vi "acquire multi waves by LAN subvi.vi"(0 "TCP Network Connection in":refnum<k5>, 5 "WFGraph Refnum":refnum<vi>, 7 "data in":string, 9 "data in":string, 11 "error in (no error)":errorcluster) -> (2 "CH1 SCALE":string, 3 "CH1 VOLTS/DIV":string, 4 "CH2 VOLTS/DIV":string, 6 "CH2 SCALE":string, 8 "CH2 PROBE":string, 10 "Waveform Graph":i32[][](graph), 13 "CH1 PROBE":string, 14 "CH2":string)   [LabVIEW 2013]
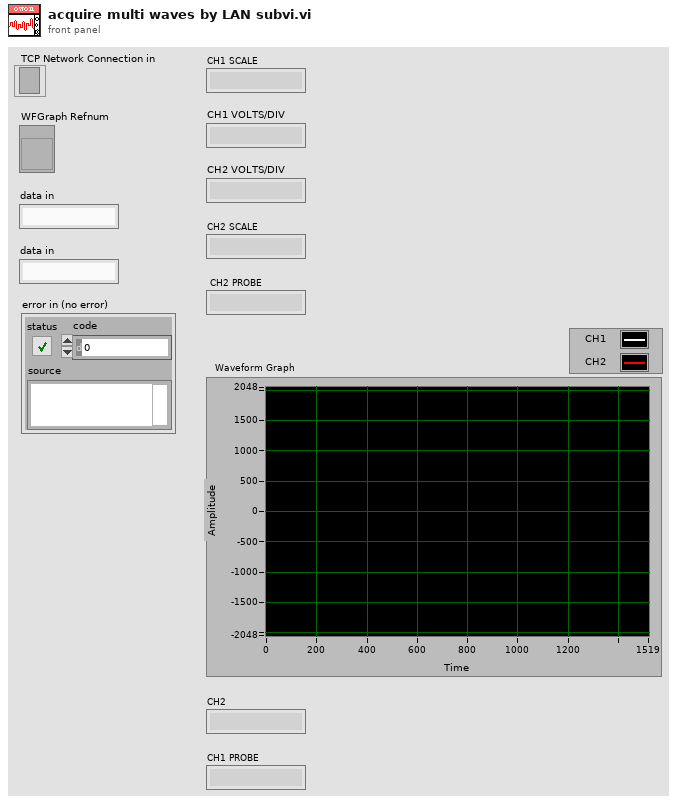
[diagram p1: front panel]
types:
  T1 = enum16{"Standard", "Buffered", "CRLF", "Immediate"}
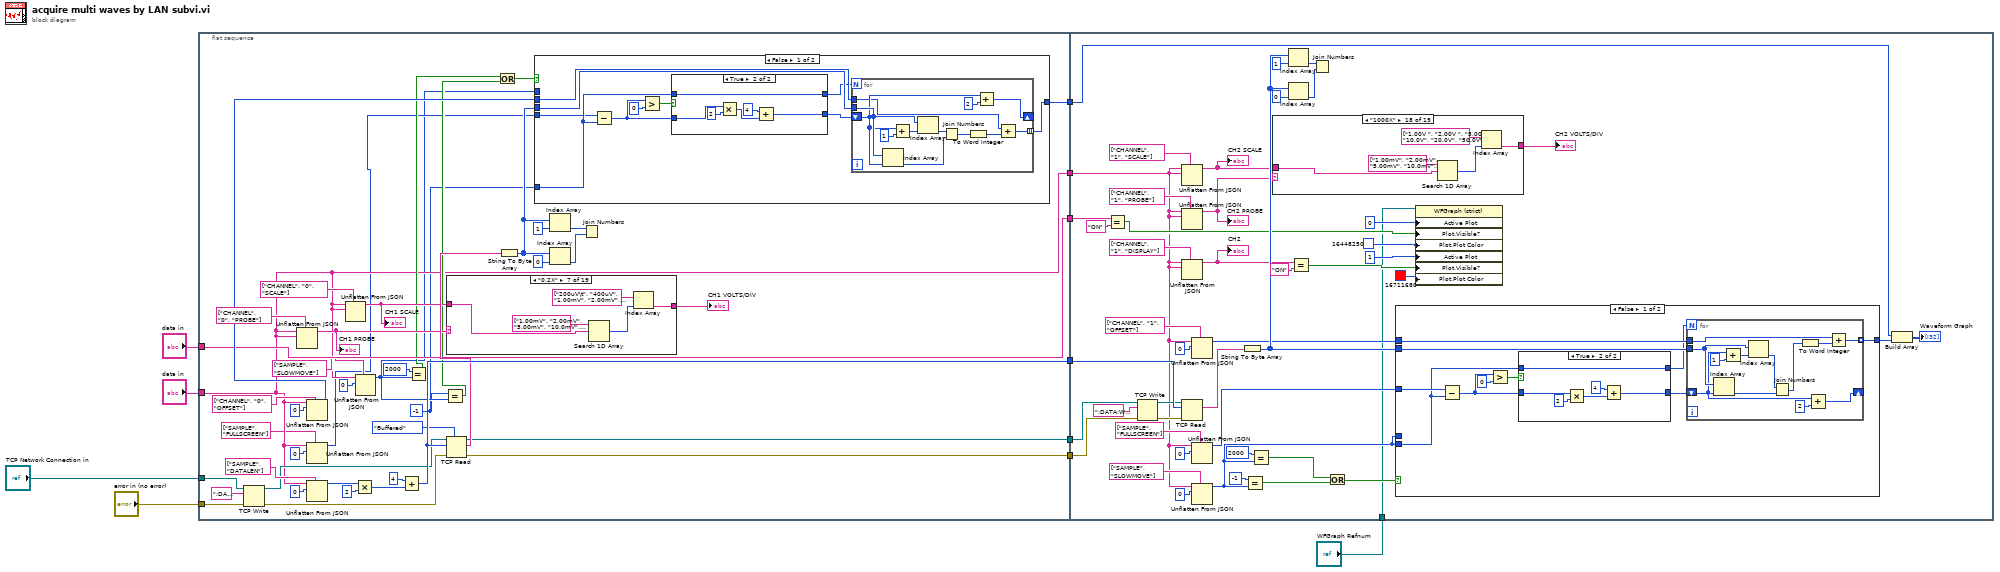
[diagram p0: block diagram]
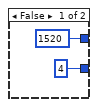
[diagram p2: hidden frame]
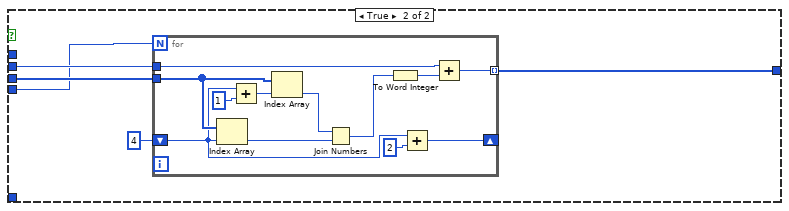
[diagram p3: hidden frame]
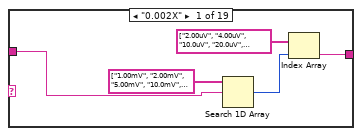
[diagram p4: hidden frame]
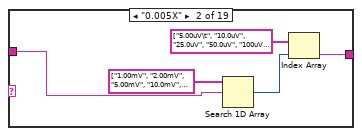
[diagram p5: hidden frame]
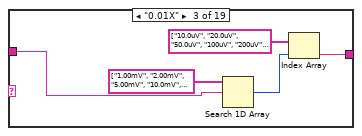
[diagram p6: hidden frame]
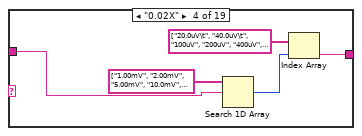
[diagram p7: hidden frame]
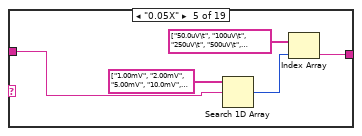
[diagram p8: hidden frame]
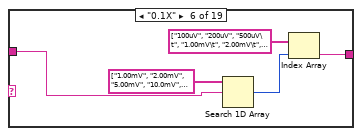
[diagram p9: hidden frame]
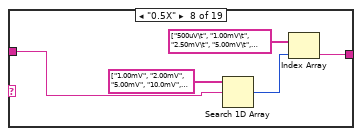
[diagram p10: hidden frame]
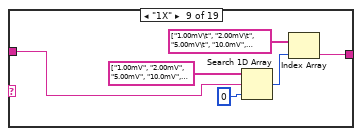
[diagram p11: hidden frame]
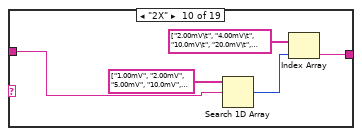
[diagram p12: hidden frame]
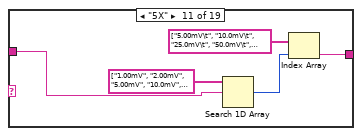
[diagram p13: hidden frame]
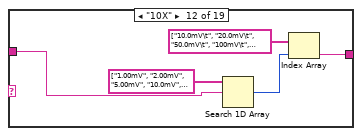
[diagram p14: hidden frame]
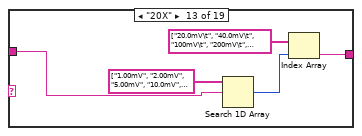
[diagram p15: hidden frame]
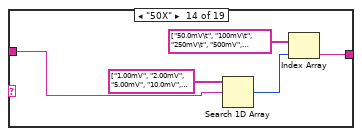
[diagram p16: hidden frame]
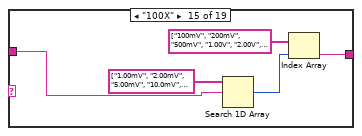
[diagram p17: hidden frame]
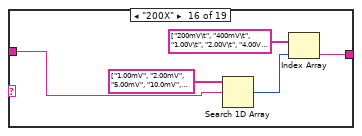
[diagram p18: hidden frame]
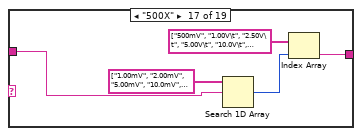
[diagram p19: hidden frame]
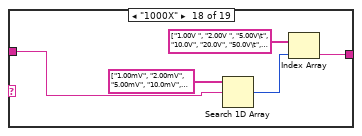
[diagram p20: hidden frame]
diagram:
  n1 = flat-sequence {
    tunnel: [w17] -> w9
    tunnel: [w34] -> w10
    tunnel: [w38] -> w11
    tunnel: "error in (no error)" -> [w36]
    tunnel: "data in" -> [w17]
    tunnel: "TCP Network Connection in" -> [w35]
    tunnel: [w29] -> w8
    tunnel: [w28] -> w7
    tunnel: [w24] -> w6
    tunnel: "data in" -> [w24]
    tunnel: w11 -> [w211]
    tunnel: w10 -> [w230]
    tunnel: w9 -> [w201]
    tunnel: w8 -> [w226]
    tunnel: w7 -> [w225]
    tunnel: w6 -> [w220]
    tunnel: "WFGraph Refnum" -> [w198]
    frame #0 {
      w12 = -1 ("x")
      n2 = TCP Write(connection ID=w35, data in=":DATA:WAVE:SCREEN:CH1?" ("ID Query"), error in (no error)=w36) -> (connection ID out=w33:refnum<k5>, error out=w32:errorcluster)  [unwired: 1 in, 1 out]
      n3 = Unflatten From JSON(path=string[] ["CHANNEL", "0", "PROBE"], JSON string=w17, type and defaults=w17) -> (value=w27:string)  [unwired: 4 in, 1 out]
      "CH1 PROBE" <- w27
      n4 = Unflatten From JSON(path=string[] ["CHANNEL", "0", "OFFSET"], JSON string=w17, type and defaults=0) -> (value=w45:i32)  [unwired: 4 in, 1 out]
      n5 = Unflatten From JSON(path=string[] ["SAMPLE", "FULLSCREEN"], JSON string=w17, type and defaults=0) -> (value=w14:i32)  [unwired: 4 in, 1 out]
      n6 = Unflatten From JSON(path=string[] ["SAMPLE", "DATALEN"], JSON string=w17, type and defaults=0) -> (value=w42:i32)  [unwired: 4 in, 1 out]
      n7 = Unflatten From JSON(path=string[] ["CHANNEL", "0", "SCALE"], JSON string=w17, type and defaults=w17) -> (value=w26:string)  [unwired: 4 in, 1 out]
      "CH1 SCALE" <- w26
      n8 = Multiply(x=w42, y=2) -> (x*y=w40:i32)
      n9 = Unflatten From JSON(path=string[] ["SAMPLE", "SLOWMOVE"], JSON string=w17, type and defaults=0) -> (value=w13:i32)  [unwired: 4 in, 1 out]
      n10 = Add(x=4, y=w40) -> (x+y=w34:i32)
      n11 = Equal?(x=2000, y=w13) -> (x = y?=w19:bool)
      n12 = Equal?(x=w12, y=w13) -> (x = y?=w20:bool)
      n13 = case shown="\"0.2X\"" w27 {
        tunnel: w26 -> [w105 w110 w115 w120 w125 w130 w135 w140 w145 w151 w156 w161 w166 w171 w176 w181 w186 w191 w197]
        tunnel: [w104 w109 w114 w119 w124 w129 w134 w139 w144 w150 w155 w160 w165 w170 w175 w180 w185 w190 w194] -> w25
        frame "0.002X" {
          n14 = Search 1D Array(1D array=string[] ["1.00mV", "2.00mV", "5.00mV", "10.0mV", "20.0mV", "50.0mV", "100mV", "200mV", "500mV", "1.00V", "2.00V", "5.00V", "10.0V", "20.0V"], element=w105) -> (index of element=w106:i32)  [unwired: 1 in]
          n15 = Index Array(array=string[] ["2.00uV", "4.00uV", "10.0uV", "20.0uV", "50.0uV", "100uV", "200uV", "400uV", "1.00mV", "2.00mV\t", "4.00mV", "10.0mV", "20.0mV", "40.0mV"], index=w106) -> (element=w104:string)
        }
        frame "0.005X" {
          n16 = Search 1D Array(1D array=string[] ["1.00mV", "2.00mV", "5.00mV", "10.0mV", "20.0mV", "50.0mV", "100mV", "200mV", "500mV", "1.00V", "2.00V", "5.00V", "10.0V", "20.0V"], element=w110) -> (index of element=w111:i32)  [unwired: 1 in]
          n17 = Index Array(array=string[] ["5.00uV\t", "10.0uV", "25.0uV", "50.0uV", "100uV", "250uV", "500uV", "1.00mV\t", "2.50mV", "5.00mV", "10.0mV", "25.0mV", "50.0mV", "100mV"], index=w111) -> (element=w109:string)
        }
        frame "0.01X" {
          n18 = Search 1D Array(1D array=string[] ["1.00mV", "2.00mV", "5.00mV", "10.0mV", "20.0mV", "50.0mV", "100mV", "200mV", "500mV", "1.00V", "2.00V", "5.00V", "10.0V", "20.0V"], element=w115) -> (index of element=w116:i32)  [unwired: 1 in]
          n19 = Index Array(array=string[] ["10.0uV", "20.0uV", "50.0uV", "100uV", "200uV", "500uV", "1.00mV\t", "2.00mV\t", "5.00mV", "10.0mV\t", "20.0mV\t", "50.0mV", "100mV", "200mV"], index=w116) -> (element=w114:string)
        }
        frame "0.02X" {
          n20 = Search 1D Array(1D array=string[] ["1.00mV", "2.00mV", "5.00mV", "10.0mV", "20.0mV", "50.0mV", "100mV", "200mV", "500mV", "1.00V", "2.00V", "5.00V", "10.0V", "20.0V"], element=w120) -> (index of element=w121:i32)  [unwired: 1 in]
          n21 = Index Array(array=string[] ["20.0uV\t", "40.0uV\t", "100uV", "200uV", "400uV", "1.00mV", "2.00mV", "4.00mV", "10.0mV", "20.0mV", "40.0mV", "100mV", "200mV", "400mV"], index=w121) -> (element=w119:string)
        }
        frame "0.05X" {
          n22 = Search 1D Array(1D array=string[] ["1.00mV", "2.00mV", "5.00mV", "10.0mV", "20.0mV", "50.0mV", "100mV", "200mV", "500mV", "1.00V", "2.00V", "5.00V", "10.0V", "20.0V"], element=w125) -> (index of element=w126:i32)  [unwired: 1 in]
          n23 = Index Array(array=string[] ["50.0uV\t", "100uV\t", "250uV\t", "500uV\t", "1.00mV", "2.50mV\t", "5.00mV\t", "10.0mV\t", "25.0mV", "50.0mV\t", "100mV", "250mV", "500mV", "1.00V"], index=w126) -> (element=w124:string)
        }
        frame "0.1X" {
          n24 = Search 1D Array(1D array=string[] ["1.00mV", "2.00mV", "5.00mV", "10.0mV", "20.0mV", "50.0mV", "100mV", "200mV", "500mV", "1.00V", "2.00V", "5.00V", "10.0V", "20.0V"], element=w130) -> (index of element=w131:i32)  [unwired: 1 in]
          n25 = Index Array(array=string[] ["100uV", "200uV", "500uV\t", "1.00mV\t", "2.00mV\t", "5.00mV\t", "10.0mV\t", "20.0mV\t", "50.0mV\t", "100mV", "200mV", "500mV\t", "1.00V", "2.00V"], index=w131) -> (element=w129:string)
        }
        frame "0.2X" {
          n26 = Search 1D Array(1D array=string[] ["1.00mV", "2.00mV", "5.00mV", "10.0mV", "20.0mV", "50.0mV", "100mV", "200mV", "500mV", "1.00V", "2.00V", "5.00V", "10.0V", "20.0V"], element=w135) -> (index of element=w136:i32)  [unwired: 1 in]
          n27 = Index Array(array=string[] ["200uV\t", "400uV", "1.00mV", "2.00mV", "4.00mV\t", "10.0mV", "20.0mV", "40.0mV\t", "100mV", "200mV", "400mV", "1.00V", "2.00V", "4.00V"], index=w136) -> (element=w134:string)
        }
        frame "0.5X" {
          n28 = Search 1D Array(1D array=string[] ["1.00mV", "2.00mV", "5.00mV", "10.0mV", "20.0mV", "50.0mV", "100mV", "200mV", "500mV", "1.00V", "2.00V", "5.00V", "10.0V", "20.0V"], element=w140) -> (index of element=w141:i32)  [unwired: 1 in]
          n29 = Index Array(array=string[] ["500uV\t", "1.00mV\t", "2.50mV\t", "5.00mV\t", "10.0mV\t", "25.0mV\t", "50.0mV\t", "100mV", "250mV\t", "500mV\t", "1.00V\t", "2.50V\t", "5.00V\t", "10.0V"], index=w141) -> (element=w139:string)
        }
        frame "1X" {
          n30 = Search 1D Array(1D array=string[] ["1.00mV", "2.00mV", "5.00mV", "10.0mV", "20.0mV", "50.0mV", "100mV", "200mV", "500mV", "1.00V", "2.00V", "5.00V", "10.0V", "20.0V"], element=w145, start index (0)=0 ("开始索引(0)")) -> (index of element=w146:i32)
          n31 = Index Array(array=string[] ["1.00mV\t", "2.00mV\t", "5.00mV\t", "10.0mV", "20.0mV", "50.0mV", "100mV", "200mV\t", "500mV", "1.00V\t", "2.00V", "5.00V", "10.0V", "20.0V"], index=w146) -> (element=w144:string)
        }
        frame "2X" {
          n32 = Search 1D Array(1D array=string[] ["1.00mV", "2.00mV", "5.00mV", "10.0mV", "20.0mV", "50.0mV", "100mV", "200mV", "500mV", "1.00V", "2.00V", "5.00V", "10.0V", "20.0V"], element=w151) -> (index of element=w152:i32)  [unwired: 1 in]
          n33 = Index Array(array=string[] ["2.00mV\t", "4.00mV\t", "10.0mV\t", "20.0mV\t", "40.0mV", "100mV\t", "200mV", "400mV", "1.00V\t", "2.00V", "4.00V", "10.0V", "20.0V", "40.0V"], index=w152) -> (element=w150:string)
        }
        frame "5X" {
          n34 = Search 1D Array(1D array=string[] ["1.00mV", "2.00mV", "5.00mV", "10.0mV", "20.0mV", "50.0mV", "100mV", "200mV", "500mV", "1.00V", "2.00V", "5.00V", "10.0V", "20.0V"], element=w156) -> (index of element=w157:i32)  [unwired: 1 in]
          n35 = Index Array(array=string[] ["5.00mV\t", "10.0mV\t", "25.0mV\t", "50.0mV\t", "100mV\t", "250mV\t", "500mV", "1.00V", "2.50V\t", "5.00V", "10.0V\t", "25.0V", "50.0V ", "100V"], index=w157) -> (element=w155:string)
        }
        frame "10X" {
          n36 = Search 1D Array(1D array=string[] ["1.00mV", "2.00mV", "5.00mV", "10.0mV", "20.0mV", "50.0mV", "100mV", "200mV", "500mV", "1.00V", "2.00V", "5.00V", "10.0V", "20.0V"], element=w161) -> (index of element=w162:i32)  [unwired: 1 in]
          n37 = Index Array(array=string[] ["10.0mV\t", "20.0mV\t", "50.0mV\t", "100mV\t", "200mV", "500mV\t", "1.00V", "2.00V\t", "5.00V\t", "10.0V\t", "20.0V\t", "50.0V", "100V ", "200V"], index=w162) -> (element=w160:string)
        }
        frame "20X" {
          n38 = Search 1D Array(1D array=string[] ["1.00mV", "2.00mV", "5.00mV", "10.0mV", "20.0mV", "50.0mV", "100mV", "200mV", "500mV", "1.00V", "2.00V", "5.00V", "10.0V", "20.0V"], element=w166) -> (index of element=w167:i32)  [unwired: 1 in]
          n39 = Index Array(array=string[] ["20.0mV\t", "40.0mV\t", "100mV\t", "200mV\t", "400mV", "1.00V\t", "2.00V\t", "4.00V\t", "10.0V\t", "20.0V\t", "40.0V", "100V", "200V\t", "400V"], index=w167) -> (element=w165:string)
        }
        frame "50X" {
          n40 = Search 1D Array(1D array=string[] ["1.00mV", "2.00mV", "5.00mV", "10.0mV", "20.0mV", "50.0mV", "100mV", "200mV", "500mV", "1.00V", "2.00V", "5.00V", "10.0V", "20.0V"], element=w171) -> (index of element=w172:i32)  [unwired: 1 in]
          n41 = Index Array(array=string[] ["50.0mV\t", "100mV\t", "250mV\t", "500mV", "1.00V", "2.50V\t", "5.00V\t", "10.0V\t", "25.0V\t", "50.0V\t", "100V", "250V", "500V\t", "1.00kV"], index=w172) -> (element=w170:string)
        }
        frame "100X" {
          n42 = Search 1D Array(1D array=string[] ["1.00mV", "2.00mV", "5.00mV", "10.0mV", "20.0mV", "50.0mV", "100mV", "200mV", "500mV", "1.00V", "2.00V", "5.00V", "10.0V", "20.0V"], element=w176) -> (index of element=w177:i32)  [unwired: 1 in]
          n43 = Index Array(array=string[] ["100mV", "200mV", "500mV", "1.00V", "2.00V", "5.00V", "10.0V", "20.0V", "50.0V", "100V   ", "200V", "500V", "1.00kV\t", "2.00kV"], index=w177) -> (element=w175:string)
        }
        frame "200X" {
          n44 = Search 1D Array(1D array=string[] ["1.00mV", "2.00mV", "5.00mV", "10.0mV", "20.0mV", "50.0mV", "100mV", "200mV", "500mV", "1.00V", "2.00V", "5.00V", "10.0V", "20.0V"], element=w181) -> (index of element=w182:i32)  [unwired: 1 in]
          n45 = Index Array(array=string[] ["200mV\t", "400mV\t", "1.00V\t", "2.00V\t", "4.00V\t", "10.0V\t", "20.0V\t", "40.0V\t", "100V   ", "200V    ", "400V   ", "1.00kV", "2.00kV", "4.00kV"], index=w182) -> (element=w180:string)
        }
        frame "500X" {
          n46 = Search 1D Array(1D array=string[] ["1.00mV", "2.00mV", "5.00mV", "10.0mV", "20.0mV", "50.0mV", "100mV", "200mV", "500mV", "1.00V", "2.00V", "5.00V", "10.0V", "20.0V"], element=w186) -> (index of element=w187:i32)  [unwired: 1 in]
          n47 = Index Array(array=string[] ["500mV", "1.00V\t", "2.50V\t", "5.00V\t", "10.0V\t", "25.0V", "50.0V", "100V   ", "250V\t", "500V\t    ", "1.00kV\t", "2.50kV", "5.00kV", "10.0kV"], index=w187) -> (element=w185:string)
        }
        frame "1000X" {
          n48 = Search 1D Array(1D array=string[] ["1.00mV", "2.00mV", "5.00mV", "10.0mV", "20.0mV", "50.0mV", "100mV", "200mV", "500mV", "1.00V", "2.00V", "5.00V", "10.0V", "20.0V"], element=w191) -> (index of element=w192:i32)  [unwired: 1 in]
          n49 = Index Array(array=string[] ["1.00V ", "2.00V ", "5.00V\t", "10.0V", "20.0V", "50.0V\t", "100V", "200V  ", "500V   ", "1.00kV\t   ", "2.00kV ", "5.00kV\t", "10.0kV", "20.0kV"], index=w192) -> (element=w190:string)
        }
        frame "0.001X", Default {
          n50 = Search 1D Array(1D array=string[] ["1.00mV", "2.00mV", "5.00mV", "10.0mV", "20.0mV", "50.0mV", "100mV", "200mV", "500mV", "1.00V", "2.00V", "5.00V", "10.0V", "20.0V"], element=w197) -> (index of element=w196:i32)  [unwired: 1 in]
          n51 = Index Array(array=string[] ["1.00uV", "2.00uV", "5.00uV", "10.0uV", "20.0uV", "50.0uV,\t", "100uV,\t", "200uV,\t", "500uV,\t", "1.00mV,\t", "2.00mV,\t", "5.00mV,\t", "10.0mV, ", "20.0mv"], index=w196) -> (element=w194:string)
        }
      }
      "CH1 VOLTS/DIV" <- w25
      n52 = TCP Read(connection ID=w33, bytes to read=w34, error in (no error)=w32, 7:T1."Buffered" ("mode (standard)")) -> (connection ID out=w29:refnum<k5>, data out=w31:string, error out=w28:errorcluster)  [unwired: 1 in]
      n53 = Or(x=w19, y=w20) -> (x .or. y?=w18:bool)
      n54 = String To Byte Array(string=w31) -> (unsigned byte array=w48:u8[])
      n55 = case shown="False" w18 {
        tunnel: w48 -> [w64 w89]
        tunnel: w45 -> [w63 w87]
        tunnel: [w62 w86] -> w38
        tunnel: w14 -> [w57 w85]
        tunnel: w13 -> [_ _]
        tunnel: w12 -> [w58 _]
        frame False {
          n56 = Subtract(x=w57, y=w58) -> (x-y=w60:i32)
          n57 = Greater?(x=w60, y=0) -> (0:w59:bool)
          n58 = case shown="True" w59 {
            tunnel: [4 w71] -> w55
            tunnel: w60 -> [_ w68]
            tunnel: [1520 w67] -> w56
            tunnel: w58 -> [_ w67]
            frame False {
            }
            frame True {
              n59 = Multiply(x=w68, y=2) -> (x*y=w70:i32)
              n60 = Add(x=4, y=w70) -> (x+y=w71:i32)
            }
          }
          n61 = for {
            N: w56 -> [_]
            tunnel: w64 -> [w84]
            shift-right: [w81] -> _
            shift-left: w55 -> [w80]
            tunnel: [w78] -> w62 mode=indexing
            tunnel: w63 -> [w75]
            n62 = Index Array(array=w84, index=w80) -> (element=w76:u8)
            n63 = Add(x=w80, y=1) -> (x+y=w83:i32)
            n64 = Index Array(array=w84, index=w83) -> (element=w77:u8)
            n65 = Join Numbers(hi=w77, lo=w76) -> ((hi.lo)=w74:u16)
            n66 = To Word Integer(number=w74) -> (16bit integer=w73:i16)
            n67 = Add(x=w80, y=2) -> (x+y=w81:i32)
            n68 = Add(x=w75, y=w73) -> (x+y=w78:i32)
          }
        }
        frame True {
          n69 = for {
            N: w85 -> [_]
            tunnel: w89 -> [w101]
            shift-right: [w98] -> _
            shift-left: 4 -> [w97]
            tunnel: [w95] -> w86 mode=indexing
            tunnel: w87 -> [w92]
            n70 = Index Array(array=w101, index=w97) -> (element=w93:u8)
            n71 = Add(x=w97, y=1) -> (x+y=w100:i32)
            n72 = Index Array(array=w101, index=w100) -> (element=w94:u8)
            n73 = Join Numbers(hi=w94, lo=w93) -> ((hi.lo)=w91:u16)
            n74 = To Word Integer(number=w91) -> (16bit integer=w90:i16)
            n75 = Add(x=w97, y=2) -> (x+y=w98:i32)
            n76 = Add(x=w92, y=w90) -> (x+y=w95:i32)
          }
        }
      }
      n77 = Index Array(array=w48, index=1) -> (element=w52:u8)
      n78 = Index Array(array=w48, index=0) -> (element=w51:u8)
      n79 = Join Numbers(hi=w52, lo=w51) -> ()  [unwired: 1 out]
    }
    frame #1 {
      n80 = Equal?(x=w220, y="ON") -> (x = y?=w221:bool)
      n81 = TCP Write(connection ID=w226, data in=":DATA:WAVE:SCREEN:CH2?" ("ID Query"), error in (no error)=w225) -> (connection ID out=w229:refnum<k5>, error out=w228:errorcluster)  [unwired: 1 in, 1 out]
      n82 = TCP Read(connection ID=w229, bytes to read=w230, error in (no error)=w228) -> (data out=w227:string)  [unwired: 2 in, 2 out]
      n83 = Unflatten From JSON(path=string[] ["CHANNEL", "1", "SCALE"], JSON string=w201, type and defaults=w201) -> (value=w224:string)  [unwired: 4 in, 1 out]
      "CH2 SCALE" <- w224
      n84 = Unflatten From JSON(path=string[] ["CHANNEL", "1", "PROBE"], JSON string=w201, type and defaults=w201) -> (value=w223:string)  [unwired: 4 in, 1 out]
      "CH2 PROBE" <- w223
      n85 = Unflatten From JSON(path=string[] ["CHANNEL", "1", "DISPLAY"], JSON string=w201, type and defaults=w201) -> (value=w214:string)  [unwired: 4 in, 1 out]
      "CH2" <- w214
      n86 = Unflatten From JSON(path=string[] ["CHANNEL", "1", "OFFSET"], JSON string=w201, type and defaults=0) -> (value=w234:i32)  [unwired: 4 in, 1 out]
      n87 = Unflatten From JSON(path=string[] ["SAMPLE", "FULLSCREEN"], JSON string=w201, type and defaults=0) -> (value=w208:i32)  [unwired: 4 in, 1 out]
      n88 = Unflatten From JSON(path=string[] ["SAMPLE", "SLOWMOVE"], JSON string=w201, type and defaults=0) -> (value=w199:i32)  [unwired: 4 in, 1 out]
      n89 = String To Byte Array(string=w227) -> (unsigned byte array=w235:u8[])
      n90 = Equal?(x=-1, y=w199) -> (x = y?=w206:bool)
      n91 = Equal?(x=2000, y=w199) -> (x = y?=w207:bool)
      n92 = case shown="\"1000X\"" w223 {
        tunnel: w224 -> [w295 w300 w305 w310 w315 w320 w325 w330 w335 w341 w346 w351 w356 w361 w366 w371 w376 w381 w387]
        tunnel: [w294 w299 w304 w309 w314 w319 w324 w329 w334 w340 w345 w350 w355 w360 w365 w370 w375 w380 w384] -> w222
        frame "0.002X" {
          n93 = Search 1D Array(1D array=string[] ["1.00mV", "2.00mV", "5.00mV", "10.0mV", "20.0mV", "50.0mV", "100mV", "200mV", "500mV", "1.00V", "2.00V", "5.00V", "10.0V", "20.0V"], element=w295) -> (index of element=w296:i32)  [unwired: 1 in]
          n94 = Index Array(array=string[] ["2.00uV", "4.00uV", "10.0uV", "20.0uV", "50.0uV", "100uV", "200uV", "400uV", "1.00mV", "2.00mV\t", "4.00mV", "10.0mV", "20.0mV", "40.0mV"], index=w296) -> (element=w294:string)
        }
        frame "0.005X" {
          n95 = Search 1D Array(1D array=string[] ["1.00mV", "2.00mV", "5.00mV", "10.0mV", "20.0mV", "50.0mV", "100mV", "200mV", "500mV", "1.00V", "2.00V", "5.00V", "10.0V", "20.0V"], element=w300) -> (index of element=w301:i32)  [unwired: 1 in]
          n96 = Index Array(array=string[] ["5.00uV\t", "10.0uV", "25.0uV", "50.0uV", "100uV", "250uV", "500uV", "1.00mV\t", "2.50mV", "5.00mV", "10.0mV", "25.0mV", "50.0mV", "100mV"], index=w301) -> (element=w299:string)
        }
        frame "0.01X" {
          n97 = Search 1D Array(1D array=string[] ["1.00mV", "2.00mV", "5.00mV", "10.0mV", "20.0mV", "50.0mV", "100mV", "200mV", "500mV", "1.00V", "2.00V", "5.00V", "10.0V", "20.0V"], element=w305) -> (index of element=w306:i32)  [unwired: 1 in]
          n98 = Index Array(array=string[] ["10.0uV", "20.0uV", "50.0uV", "100uV", "200uV", "500uV", "1.00mV\t", "2.00mV\t", "5.00mV", "10.0mV\t", "20.0mV\t", "50.0mV", "100mV", "200mV"], index=w306) -> (element=w304:string)
        }
        frame "0.02X" {
          n99 = Search 1D Array(1D array=string[] ["1.00mV", "2.00mV", "5.00mV", "10.0mV", "20.0mV", "50.0mV", "100mV", "200mV", "500mV", "1.00V", "2.00V", "5.00V", "10.0V", "20.0V"], element=w310) -> (index of element=w311:i32)  [unwired: 1 in]
          n100 = Index Array(array=string[] ["20.0uV\t", "40.0uV\t", "100uV", "200uV", "400uV", "1.00mV", "2.00mV", "4.00mV", "10.0mV", "20.0mV", "40.0mV", "100mV", "200mV", "400mV"], index=w311) -> (element=w309:string)
        }
        frame "0.05X" {
          n101 = Search 1D Array(1D array=string[] ["1.00mV", "2.00mV", "5.00mV", "10.0mV", "20.0mV", "50.0mV", "100mV", "200mV", "500mV", "1.00V", "2.00V", "5.00V", "10.0V", "20.0V"], element=w315) -> (index of element=w316:i32)  [unwired: 1 in]
          n102 = Index Array(array=string[] ["50.0uV\t", "100uV\t", "250uV\t", "500uV\t", "1.00mV", "2.50mV\t", "5.00mV\t", "10.0mV\t", "25.0mV", "50.0mV\t", "100mV", "250mV", "500mV", "1.00V"], index=w316) -> (element=w314:string)
        }
        frame "0.1X" {
          n103 = Search 1D Array(1D array=string[] ["1.00mV", "2.00mV", "5.00mV", "10.0mV", "20.0mV", "50.0mV", "100mV", "200mV", "500mV", "1.00V", "2.00V", "5.00V", "10.0V", "20.0V"], element=w320) -> (index of element=w321:i32)  [unwired: 1 in]
          n104 = Index Array(array=string[] ["100uV", "200uV", "500uV\t", "1.00mV\t", "2.00mV\t", "5.00mV\t", "10.0mV\t", "20.0mV\t", "50.0mV\t", "100mV", "200mV", "500mV\t", "1.00V", "2.00V"], index=w321) -> (element=w319:string)
        }
        frame "0.2X" {
          n105 = Search 1D Array(1D array=string[] ["1.00mV", "2.00mV", "5.00mV", "10.0mV", "20.0mV", "50.0mV", "100mV", "200mV", "500mV", "1.00V", "2.00V", "5.00V", "10.0V", "20.0V"], element=w325) -> (index of element=w326:i32)  [unwired: 1 in]
          n106 = Index Array(array=string[] ["200uV\t", "400uV", "1.00mV", "2.00mV", "4.00mV\t", "10.0mV", "20.0mV", "40.0mV\t", "100mV", "200mV", "400mV", "1.00V", "2.00V", "4.00V"], index=w326) -> (element=w324:string)
        }
        frame "0.5X" {
          n107 = Search 1D Array(1D array=string[] ["1.00mV", "2.00mV", "5.00mV", "10.0mV", "20.0mV", "50.0mV", "100mV", "200mV", "500mV", "1.00V", "2.00V", "5.00V", "10.0V", "20.0V"], element=w330) -> (index of element=w331:i32)  [unwired: 1 in]
          n108 = Index Array(array=string[] ["500uV\t", "1.00mV\t", "2.50mV\t", "5.00mV\t", "10.0mV\t", "25.0mV\t", "50.0mV\t", "100mV", "250mV\t", "500mV\t", "1.00V\t", "2.50V\t", "5.00V\t", "10.0V"], index=w331) -> (element=w329:string)
        }
        frame "1X" {
          n109 = Search 1D Array(1D array=string[] ["1.00mV", "2.00mV", "5.00mV", "10.0mV", "20.0mV", "50.0mV", "100mV", "200mV", "500mV", "1.00V", "2.00V", "5.00V", "10.0V", "20.0V"], element=w335, start index (0)=0 ("开始索引(0)")) -> (index of element=w336:i32)
          n110 = Index Array(array=string[] ["1.00mV\t", "2.00mV\t", "5.00mV\t", "10.0mV", "20.0mV", "50.0mV", "100mV", "200mV\t", "500mV", "1.00V\t", "2.00V", "5.00V", "10.0V", "20.0V"], index=w336) -> (element=w334:string)
        }
        frame "2X" {
          n111 = Search 1D Array(1D array=string[] ["1.00mV", "2.00mV", "5.00mV", "10.0mV", "20.0mV", "50.0mV", "100mV", "200mV", "500mV", "1.00V", "2.00V", "5.00V", "10.0V", "20.0V"], element=w341) -> (index of element=w342:i32)  [unwired: 1 in]
          n112 = Index Array(array=string[] ["2.00mV\t", "4.00mV\t", "10.0mV\t", "20.0mV\t", "40.0mV", "100mV\t", "200mV", "400mV", "1.00V\t", "2.00V", "4.00V", "10.0V", "20.0V", "40.0V"], index=w342) -> (element=w340:string)
        }
        frame "5X" {
          n113 = Search 1D Array(1D array=string[] ["1.00mV", "2.00mV", "5.00mV", "10.0mV", "20.0mV", "50.0mV", "100mV", "200mV", "500mV", "1.00V", "2.00V", "5.00V", "10.0V", "20.0V"], element=w346) -> (index of element=w347:i32)  [unwired: 1 in]
          n114 = Index Array(array=string[] ["5.00mV\t", "10.0mV\t", "25.0mV\t", "50.0mV\t", "100mV\t", "250mV\t", "500mV", "1.00V", "2.50V\t", "5.00V", "10.0V\t", "25.0V", "50.0V ", "100V"], index=w347) -> (element=w345:string)
        }
        frame "10X" {
          n115 = Search 1D Array(1D array=string[] ["1.00mV", "2.00mV", "5.00mV", "10.0mV", "20.0mV", "50.0mV", "100mV", "200mV", "500mV", "1.00V", "2.00V", "5.00V", "10.0V", "20.0V"], element=w351) -> (index of element=w352:i32)  [unwired: 1 in]
          n116 = Index Array(array=string[] ["10.0mV\t", "20.0mV\t", "50.0mV\t", "100mV\t", "200mV", "500mV\t", "1.00V", "2.00V\t", "5.00V\t", "10.0V\t", "20.0V\t", "50.0V", "100V ", "200V"], index=w352) -> (element=w350:string)
        }
        frame "20X" {
          n117 = Search 1D Array(1D array=string[] ["1.00mV", "2.00mV", "5.00mV", "10.0mV", "20.0mV", "50.0mV", "100mV", "200mV", "500mV", "1.00V", "2.00V", "5.00V", "10.0V", "20.0V"], element=w356) -> (index of element=w357:i32)  [unwired: 1 in]
          n118 = Index Array(array=string[] ["20.0mV\t", "40.0mV\t", "100mV\t", "200mV\t", "400mV", "1.00V\t", "2.00V\t", "4.00V\t", "10.0V\t", "20.0V\t", "40.0V", "100V", "200V\t", "400V"], index=w357) -> (element=w355:string)
        }
        frame "50X" {
          n119 = Search 1D Array(1D array=string[] ["1.00mV", "2.00mV", "5.00mV", "10.0mV", "20.0mV", "50.0mV", "100mV", "200mV", "500mV", "1.00V", "2.00V", "5.00V", "10.0V", "20.0V"], element=w361) -> (index of element=w362:i32)  [unwired: 1 in]
          n120 = Index Array(array=string[] ["50.0mV\t", "100mV\t", "250mV\t", "500mV", "1.00V", "2.50V\t", "5.00V\t", "10.0V\t", "25.0V\t", "50.0V\t", "100V", "250V", "500V\t", "1.00kV"], index=w362) -> (element=w360:string)
        }
        frame "100X" {
          n121 = Search 1D Array(1D array=string[] ["1.00mV", "2.00mV", "5.00mV", "10.0mV", "20.0mV", "50.0mV", "100mV", "200mV", "500mV", "1.00V", "2.00V", "5.00V", "10.0V", "20.0V"], element=w366) -> (index of element=w367:i32)  [unwired: 1 in]
          n122 = Index Array(array=string[] ["100mV", "200mV", "500mV", "1.00V", "2.00V", "5.00V", "10.0V", "20.0V", "50.0V", "100V   ", "200V", "500V", "1.00kV\t", "2.00kV"], index=w367) -> (element=w365:string)
        }
        frame "200X" {
          n123 = Search 1D Array(1D array=string[] ["1.00mV", "2.00mV", "5.00mV", "10.0mV", "20.0mV", "50.0mV", "100mV", "200mV", "500mV", "1.00V", "2.00V", "5.00V", "10.0V", "20.0V"], element=w371) -> (index of element=w372:i32)  [unwired: 1 in]
          n124 = Index Array(array=string[] ["200mV\t", "400mV\t", "1.00V\t", "2.00V\t", "4.00V\t", "10.0V\t", "20.0V\t", "40.0V\t", "100V   ", "200V    ", "400V   ", "1.00kV", "2.00kV", "4.00kV"], index=w372) -> (element=w370:string)
        }
        frame "500X" {
          n125 = Search 1D Array(1D array=string[] ["1.00mV", "2.00mV", "5.00mV", "10.0mV", "20.0mV", "50.0mV", "100mV", "200mV", "500mV", "1.00V", "2.00V", "5.00V", "10.0V", "20.0V"], element=w376) -> (index of element=w377:i32)  [unwired: 1 in]
          n126 = Index Array(array=string[] ["500mV", "1.00V\t", "2.50V\t", "5.00V\t", "10.0V\t", "25.0V", "50.0V", "100V   ", "250V\t", "500V\t    ", "1.00kV\t", "2.50kV", "5.00kV", "10.0kV"], index=w377) -> (element=w375:string)
        }
        frame "1000X" {
          n127 = Search 1D Array(1D array=string[] ["1.00mV", "2.00mV", "5.00mV", "10.0mV", "20.0mV", "50.0mV", "100mV", "200mV", "500mV", "1.00V", "2.00V", "5.00V", "10.0V", "20.0V"], element=w381) -> (index of element=w382:i32)  [unwired: 1 in]
          n128 = Index Array(array=string[] ["1.00V ", "2.00V ", "5.00V\t", "10.0V", "20.0V", "50.0V\t", "100V", "200V  ", "500V   ", "1.00kV\t   ", "2.00kV ", "5.00kV\t", "10.0kV", "20.0kV"], index=w382) -> (element=w380:string)
        }
        frame "0.001X", Default {
          n129 = Search 1D Array(1D array=string[] ["1.00mV", "2.00mV", "5.00mV", "10.0mV", "20.0mV", "50.0mV", "100mV", "200mV", "500mV", "1.00V", "2.00V", "5.00V", "10.0V", "20.0V"], element=w387) -> (index of element=w386:i32)  [unwired: 1 in]
          n130 = Index Array(array=string[] ["1.00uV", "2.00uV", "5.00uV", "10.0uV", "20.0uV", "50.0uV,\t", "100uV,\t", "200uV,\t", "500uV,\t", "1.00mV,\t", "2.00mV,\t", "5.00mV,\t", "10.0mV, ", "20.0mv"], index=w386) -> (element=w384:string)
        }
      }
      "CH2 VOLTS/DIV" <- w222
      n131 = Index Array(array=w235, index=1) -> (element=w237:u8)
      n132 = Index Array(array=w235, index=0) -> (element=w236:u8)
      n133 = Equal?(x=w214, y="ON") -> (x = y?=w216:bool)
      n134 = Join Numbers(hi=w237, lo=w236) -> ()  [unwired: 1 out]
      n135 = Or(x=w207, y=w206) -> (x .or. y?=w202:bool)
      n136 = case shown="False" w202 {
        tunnel: w235 -> [w254 w279]
        tunnel: w234 -> [w253 w277]
        tunnel: [w252 w276] -> w233
        tunnel: w208 -> [w248 w275]
        tunnel: w199 -> [_ _]
        tunnel: w199 -> [w247 _]
        frame False {
          n137 = Subtract(x=w248, y=w247) -> (x-y=w250:i32)
          n138 = Greater?(x=w250, y=0) -> (0:w249:bool)
          n139 = case shown="True" w249 {
            tunnel: [4 w261] -> w245
            tunnel: w250 -> [_ w258]
            tunnel: [1520 w257] -> w246
            tunnel: w247 -> [_ w257]
            frame False {
            }
            frame True {
              n140 = Multiply(x=w258, y=2) -> (x*y=w260:i32)
              n141 = Add(x=4, y=w260) -> (x+y=w261:i32)
            }
          }
          n142 = for {
            N: w246 -> [_]
            tunnel: w254 -> [w274]
            shift-right: [w271] -> _
            shift-left: w245 -> [w270]
            tunnel: [w268] -> w252 mode=indexing
            tunnel: w253 -> [w265]
            n143 = Index Array(array=w274, index=w270) -> (element=w266:u8)
            n144 = Add(x=w270, y=1) -> (x+y=w273:i32)
            n145 = Index Array(array=w274, index=w273) -> (element=w267:u8)
            n146 = Join Numbers(hi=w267, lo=w266) -> ((hi.lo)=w264:u16)
            n147 = To Word Integer(number=w264) -> (16bit integer=w263:i16)
            n148 = Add(x=w270, y=2) -> (x+y=w271:i32)
            n149 = Add(x=w265, y=w263) -> (x+y=w268:i32)
          }
        }
        frame True {
          n150 = for {
            N: w275 -> [_]
            tunnel: w279 -> [w291]
            shift-right: [w288] -> _
            shift-left: 4 -> [w287]
            tunnel: [w285] -> w276 mode=indexing
            tunnel: w277 -> [w282]
            n151 = Index Array(array=w291, index=w287) -> (element=w283:u8)
            n152 = Add(x=w287, y=1) -> (x+y=w290:i32)
            n153 = Index Array(array=w291, index=w290) -> (element=w284:u8)
            n154 = Join Numbers(hi=w284, lo=w283) -> ((hi.lo)=w281:u16)
            n155 = To Word Integer(number=w281) -> (16bit integer=w280:i16)
            n156 = Add(x=w287, y=2) -> (x+y=w288:i32)
            n157 = Add(x=w282, y=w280) -> (x+y=w285:i32)
          }
        }
      }
      n158 = property on="Property Node" class="WFGraph (strict)"(reference=w198, "Active Plot"=u32 0 ("活动曲线"), "Plot.Visible?"=w221, "Plot.Plot Color"=u32 16448250, "Active Plot"=u32 1 ("活动曲线"), "Plot.Visible?"=w216, "Plot.Plot Color"=u32 16711680) -> ()  [unwired: 1 in, 2 out]
      n159 = Build Array(w211, w233) -> (→"Waveform Graph":i32[][])
    }
  }
